vi "Centauro Button Press.vi"(0 "GEA2 Reference In":refnum<k24>, 1 "Standalone?":bool, 5 "Button Press":enum16{"StartButtonPress", "DeepRinseKeyPress"}(ring), 7 "Press & Hold?":bool, 9 "Delay Time (s)":dbl=0.4 format="%#_13g", 11 "Error In":errorcluster) -> (4 "GEA2 Reference_ Out":refnum<k24>, 15 "Error Out":errorcluster)   [LabVIEW 2016, in "Centauro.lvlib"]
uses:
  Projects/Centauro.lvlib
  Q:/Common/DLLs/GEA3/GeaCommunication.dll
  Common/DLLs/GEA3/GeaCommunication.dll
  Tools/Laundry/Centauro Tool/Centauro Tool Support/type defs/Event Sequence.ctl
  Common/LabVIEW GEA2 Toolkit/LabVIEW_GEA2_Toolkit.lvlibp/type defs/Source_Destination.ctl
  Common/LabVIEW GEA2 Toolkit/LabVIEW_GEA2_Toolkit.lvlibp
panel:
  in  "Event ID":T1
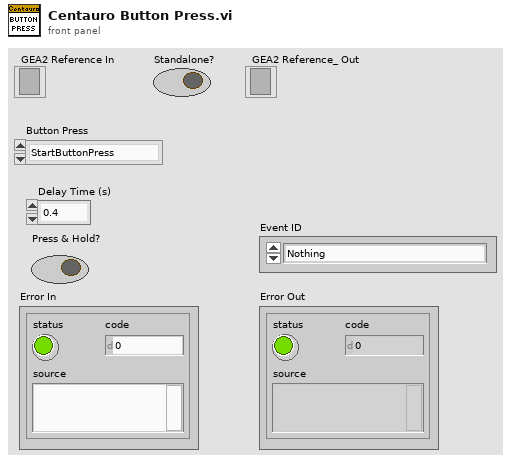
[diagram p1: front panel]
types:
  T1 = typedef "Event Sequence.ctl" = enum16{"Nothing", "StartButtonPress", "StartButtonRelease", "DeepRinseKeyPress", "DeepRinseKeyRelease", "CycleKnobPosition0", "CycleKnobPosition1", "CycleKnobPosition2", "CycleKnobPosition3", "CycleKnobPosition4", "CycleKnobPosition5", "CycleKnobPosition6", "CycleKnobPosition7", "CycleKnobPosition8", "CycleKnobPosition9", "CycleKnobPosition10", "CycleKnobPosition11", "OptionKnob1Position0", "OptionKnob1Position1", "OptionKnob1Position2", "OptionKnob1Position3", "OptionKnob1Position4", "OptionKnob1Position5", "OptionKnob2Position0", "OptionKnob2Position1", "OptionKnob2Position2", "OptionKnob2Position3", "OptionKnob2Position4"}
  T2 = typedef "LabVIEW_GEA2_Toolkit.lvlibp/Source_Destination.ctl" = cluster{"Source":u8, "Destination":u8}
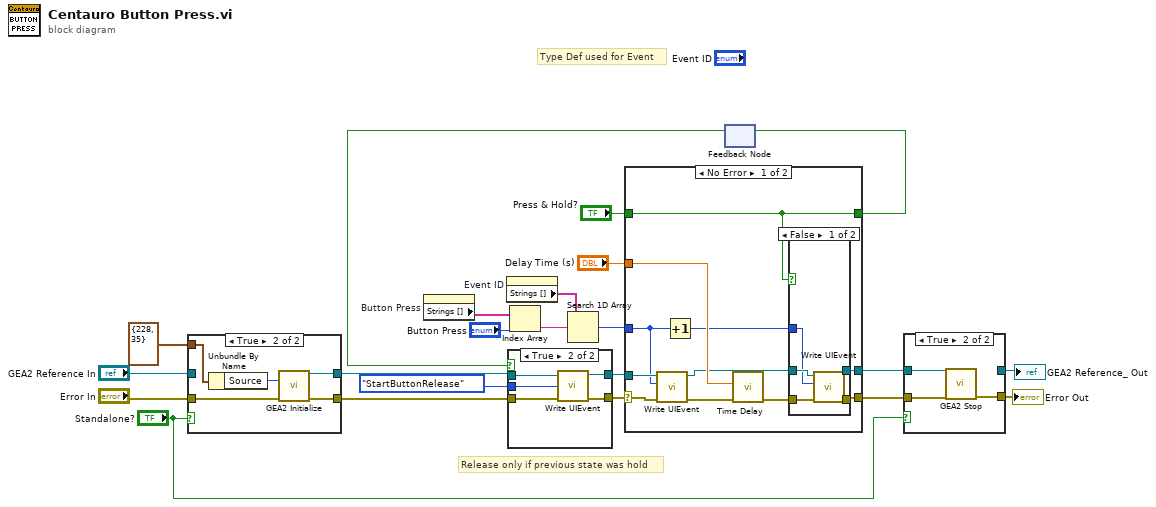
[diagram p0: block diagram]
diagram:
  # "Release only if previous state was hold"
  # "Type Def used for Event"
  n1 = case shown="True" "Standalone?" {
    tunnel: "Error In" -> [w23 w29]
    tunnel: [w23 w28] -> w10
    tunnel: "GEA2 Reference In" -> [w24 _]
    tunnel: [w24 w27] -> w6
    tunnel: T2 {"Source"=228, "Destination"=35} ("GEA Inputs") -> [_ w25]
    frame False {
    }
    frame True {
      n2 = Unbundle By Name(w25) -> ("Source"=w26:u8)
      n3 = call "GEA2 Initialize.vi"("Source Address"=w26, "error in"=w29) -> ("GEA2 Reference Out"=w27:refnum<k24>, "error out"=w28:errorcluster)  [unwired: 11 in, 1 out]
    }
  }
  n4 = property on="Button Press" class="Enum (strict)"() -> ("Strings []"=w18:string[])  [unwired: 2 in, 2 out]
  n5 = property on="Event ID" class="Enum (strict)"() -> ("Strings []"=w21:string[])  [unwired: 2 in, 2 out]
  n6 = Index Array(array=w18, index="Button Press") -> (element=w22:string)
  n7 = Search 1D Array(1D array=w21, element=w22) -> (index of element=w20:i32)  [unwired: 1 in]
  n8 = feedback #1() -> (w14:bool)  [unwired: 1 in]
  n9 = case shown="True" w14 {
    tunnel: w6 -> [w31 w36]
    tunnel: [w31 w35] -> w13
    tunnel: Event_Sequence."StartButtonRelease" ("Event ID") -> [_ w34]
    tunnel: w10 -> [w30 w33]
    tunnel: [w30 w32] -> w11
    frame False {
    }
    frame True {
      n10 = call "Write UIEvent.vi"("Error In"=w33, "Event ID"=w34, "GEA2 Reference In"=w36) -> ("Error Out"=w32:errorcluster, "GEA2 Reference Out"=w35:refnum<k24>)  [unwired: 7 in]
    }
  }
  n11 = case shown="No Error" w11 {
    selector: w11 -> [w47 w57]
    tunnel: [w42 w57] -> w4
    tunnel: w13 -> [w46 w56]
    tunnel: [w41 w56] -> w5
    tunnel: w20 -> [w38 _]
    tunnel: "Delay Time (s)" -> [w44 _]
    tunnel: "Press & Hold?" -> [w37 w55]
    tunnel: [w37 w55] -> w15
    frame No Error {
      n12 = call "Write UIEvent.vi"("Error In"=w47, "Event ID"=w38, "GEA2 Reference In"=w46) -> ("Error Out"=w45:errorcluster, "GEA2 Reference Out"=w40:refnum<k24>)  [unwired: 7 in]
      n13 = Increment(x=w38) -> (x+1=w39:i32)
      n14 = call "Time Delay"("error in (no error)"=w45, "Delay Time (s)"=w44) -> ("error out"=w43:errorcluster)  [unwired: 9 in]
      n15 = case shown="False" w37 {
        tunnel: w43 -> [w52 w53]
        tunnel: [w51 w53] -> w42
        tunnel: [w50 w54] -> w41
        tunnel: w40 -> [w49 w54]
        tunnel: w39 -> [w48 _]
        frame False {
          n16 = call "Write UIEvent.vi"("Error In"=w52, "Event ID"=w48, "GEA2 Reference In"=w49) -> ("Error Out"=w51:errorcluster, "GEA2 Reference Out"=w50:refnum<k24>)  [unwired: 7 in]
        }
        frame True {
        }
      }
    }
    frame Error {
    }
  }
  n17 = feedback-in #1(w15) -> ()
  n18 = case shown="True" "Standalone?" {
    tunnel: w5 -> [w59 w62]
    tunnel: w4 -> [w58 w61]
    tunnel: [w58 w60] -> w2
    tunnel: [w59 _] -> w1
    frame False {
    }
    frame True {
      n19 = call "GEA2 Stop.vi"("GEA2 Reference In"=w62, "Error In"=w61) -> ("Error Out"=w60:errorcluster)  [unwired: 13 in]
    }
  }
  "Error Out" <- w2
  "GEA2 Reference_ Out" <- w1
